vi "GLOBAL_QDC_Data.vi"(3 "Module":string="QDC Data", 4 "State":enum16{"Initialise", "Write", "Read"}(ring), 5 "Input Data":T1[](array[typedef])) -> (1 "Valid Read?":bool, 2 "Data Out":T1[](array[typedef]))   [LabVIEW 2014]
uses:
  QDCDataCluster.ctl
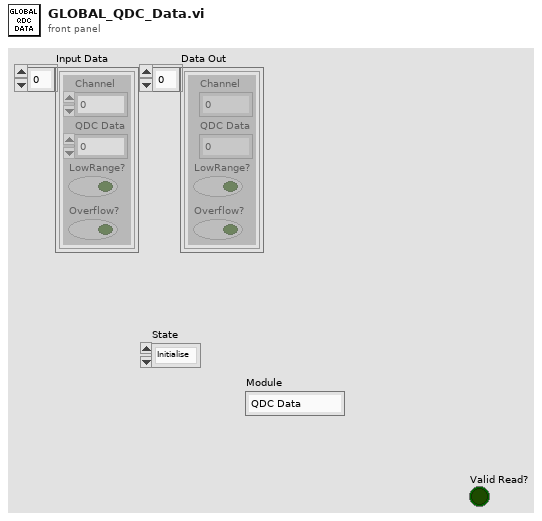
[diagram p1: front panel]
types:
  T1 = typedef "QDCDataCluster.ctl" = cluster{"Channel":u8, "QDC Data":sgl, "LowRange?":bool, "Overflow?":bool}
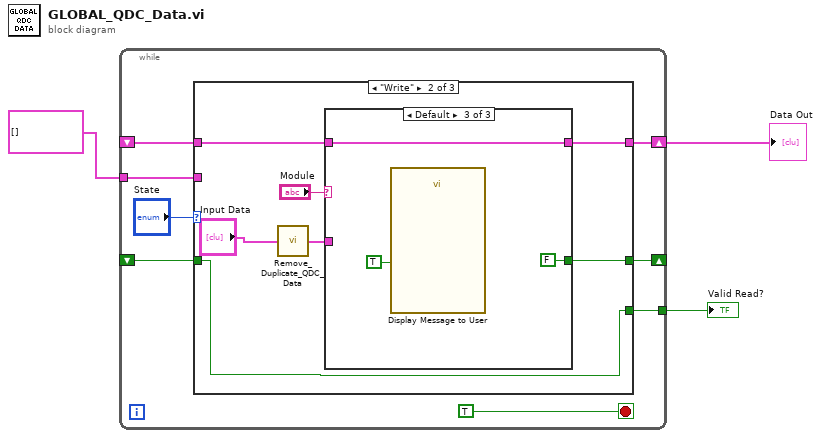
[diagram p0: block diagram]
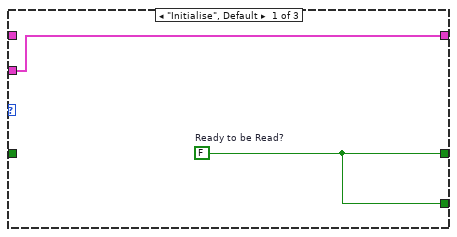
[diagram p2: hidden frame]
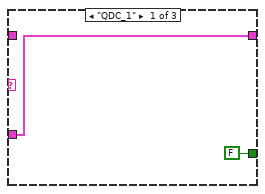
[diagram p3: hidden frame]
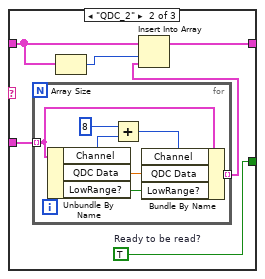
[diagram p4: hidden frame]
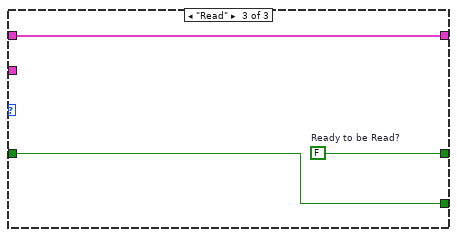
[diagram p5: hidden frame]
diagram:
  n1 = while {
    shift-right: [w5] -> w1
    shift-left: _ -> [w10]
    shift-right: [w8] -> _
    shift-left: _ -> [w7]
    tunnel: [w6] -> w3
    tunnel: T1[] [] ("appended array") -> [w4]
    stop <- TRUE stop-if-true
    n2 = case shown="\"Write\"" "State" {
      tunnel: [w12 w18 w40] -> w5
      tunnel: w10 -> [_ w19 w40]
      tunnel: [w13 w20 w41] -> w8
      tunnel: w7 -> [_ w15 w39]
      tunnel: [w13 w15 w39] -> w6
      tunnel: w4 -> [w12 _ _]
      frame "Initialise", Default {
        w13 = FALSE  # Ready to be Read?
      }
      frame "Write" {
        n3 = call "Remove_Duplicate_QDC_Data.vi"("Input Data"="Input Data") -> ("Output Data"=w16:T1[])
        n4 = case shown="Default" "Module" {
          tunnel: [FALSE ("Ready to be read?") w25 FALSE ("Ready to be read?")] -> w20
          tunnel: [w22 w28 w38] -> w18
          tunnel: w19 -> [_ w23 w38]
          tunnel: w16 -> [w22 w24 _]
          frame "QDC_1" {
          }
          frame "QDC_2" {
            w25 = TRUE  # Ready to be read?
            n5 = for {
              tunnel: w24 -> [w35] mode=indexing
              tunnel: [w29] -> w26 mode=indexing
              n6 = Unbundle By Name(w35) -> ("Channel"=w34:u8, "QDC Data"=w31:sgl, "LowRange?"=w30:bool)
              n7 = Add(x=u8 8, y=w34) -> (x+y=w33:u8)
              n8 = Bundle By Name(cluster=w35, "Channel"=w33, "QDC Data"=w31, "LowRange?"=w30) -> (w29:T1)
            }
            n9 = Array Size(array=w23) -> (size(s)=w27:i32)
            n10 = Insert Into Array(array=w23, index=w27, new element=w26) -> (w28:T1[])
          }
          frame Default {
            n11 = call "Display Message to User"("Enable"=TRUE) -> ()  [unwired: 9 in, 2 out]
          }
        }
      }
      frame "Read" {
        w41 = FALSE  # Ready to be Read?
      }
    }
  }
  "Valid Read?" <- w3
  "Data Out" <- w1
